vi "Main.vi"() -> ()   [LabVIEW 2013]
doc: "Configures a sweep and takes voltage and current readings at each point."
uses:
  <instrlib>/Keithley 24XX/Public/Data/Read (Multiple Points).vi
  <vilib>/Utility/file.llb/Read From Spreadsheet File (DBL).vi
  <instrlib>/Keithley 24XX/Keithley 24XX.lvlib
  <vilib>/gmath/NI_Gmath.lvlib
panel:
  in  "定标文件":string(combo)
  in  "Source Mode  (0: Voltage)":u16(ring) items=["Voltage", "Current"]
  in  "Serial Configuration":T1={"Baud Rate"=9600, "Parity"=0, "Data Bits"=8, "Stop Bits"=10, "Flow Control"=0} {"Flow Control" items=["None", "XON/XOFF", "RTS/CTS", "XON/XOFF & RTS/CTS", "DTR/DSR", "XON/XOFF & DTR/DSR"]; "Stop Bits" items=["1.0"=10, "1.5"=15, "2.0"=20]; "Data Bits" items=["7"=7, "8"=8]; "Parity" items=["None", "Odd", "Even", "Mark", "Space"]; "Baud Rate" items=["300"=300, "600"=600, "1200"=1200, "2400"=2400, "4800"=4800, "9600"=9600, "19200"=19200]}
  in  "VISA resource name":refnum<visa-resource-name>
  out "Waveform Graph":dbl[](graph)
  in  "Timeout (10000 ms)":i32=10000 format="%#.6g"
  in  "Maximum Amplitude (2)":dbl=2.0
  in  "Minimum Amplitude (1)":dbl=1.0
  in  "Number of Points (5)":u32=5
  in  "Compliance  Level (0.1)":dbl=0.1
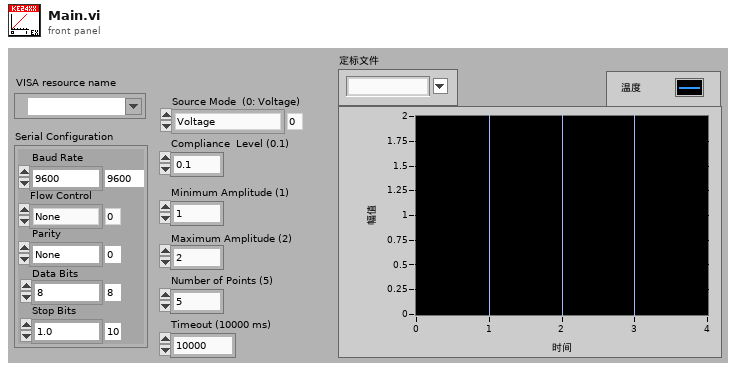
[diagram p1: front panel]
types:
  T1 = cluster{"Baud Rate":u32, "Parity":u16, "Data Bits":u16, "Stop Bits":u16, "Flow Control":u16}
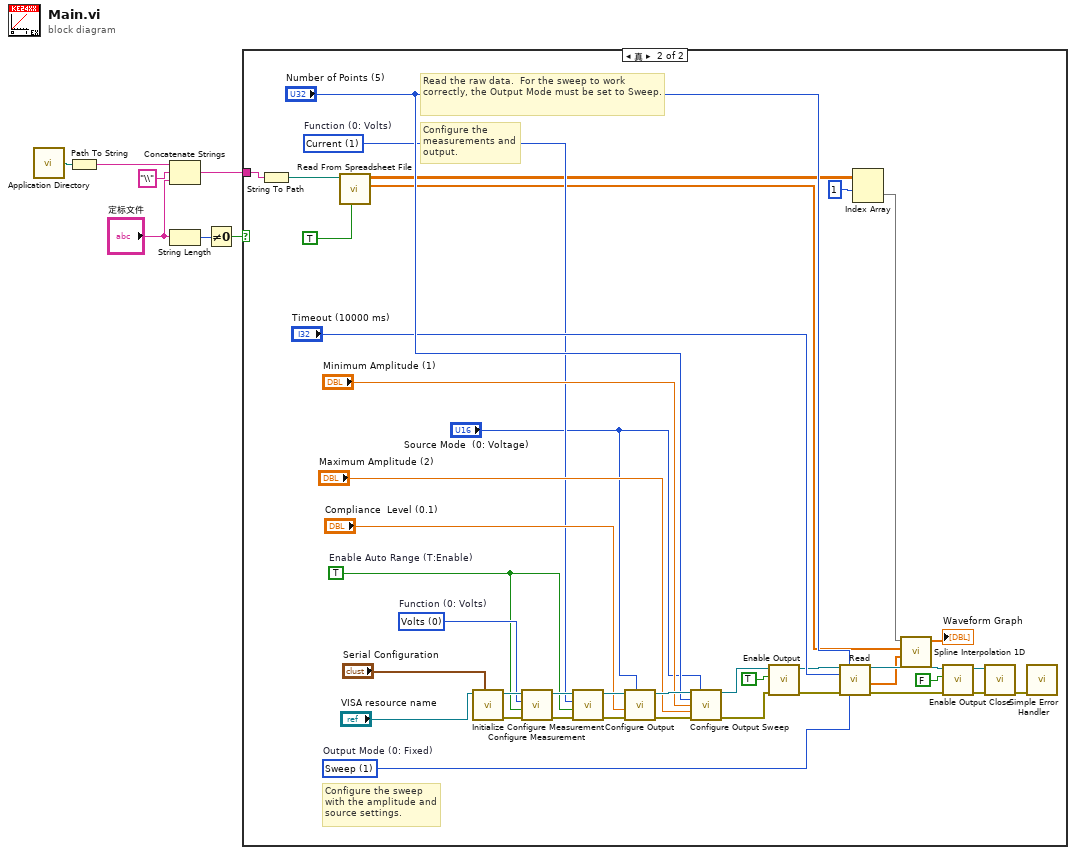
[diagram p0: block diagram]
diagram:
  n1 = call <vilib>:"Application Directory.vi"() -> ("Application Directory"=w7:path)
  n2 = Path To String(path=w7) -> (string=w6:string)
  n3 = Concatenate Strings(w6, "\\", "定标文件") -> (w2:string)
  n4 = String Length(string="定标文件") -> (length=w3:i32)
  n5 = Not Equal To 0?(x=w3) -> (x != 0?=w1:bool)
  n6 = case shown="真" w1 {
    tunnel: w2 -> [_ w9]
    frame False {
    }
    frame True {
      w19 = TRUE  # Enable Auto Range (T:Enable)
      w20 = u16 1 items=["Volts", "Current", "Resistance"]  # Function (0: Volts)
      w21 = u16 0 items=["Volts", "Current", "Resistance"]  # Function (0: Volts)
      w33 = u16 1 items=["Fixed", "Sweep", "List"]  # Output Mode (0: Fixed)
      # "Read the raw data.  For the sweep to work correctly, the Output Mode must be set to Sweep."
      # "Configure the sweep with the amplitude and source settings."
      # "Configure the measurements and output."
      n7 = String To Path(string=w9) -> (path=w8:path)
      n8 = call-poly <vilib>:"Read From Spreadsheet File.vi"("transpose (no:F)"=TRUE, "file path (dialog if empty)"=w8) -> ("first row"=w12:dbl[], "all rows"=w11:dbl[][])  [unwired: 5 in, 3 out]
      n9 = call <instrlib>:"Initialize.vi"("Serial Configuration"="Serial Configuration", "VISA resource name"="VISA resource name") -> ("error out"=w46:errorcluster, "VISA resource name out"=w47:refnum<visa-resource-name>)  [unwired: 8 in]
      n10 = call <instrlib>:"Configure Measurement.vi"("error in (no error)"=w46, "Enable Auto Range (T:Enable)"=w19, "Function (0: Volts)"=w21, "VISA resource name"=w47) -> ("error out"=w45:errorcluster, "VISA resource name out"=w44:refnum<visa-resource-name>)  [unwired: 6 in]
      n11 = call <instrlib>:"Configure Measurement.vi"("error in (no error)"=w45, "Enable Auto Range (T:Enable)"=w19, "Function (0: Volts)"=w20, "VISA resource name"=w44) -> ("error out"=w42:errorcluster, "VISA resource name out"=w43:refnum<visa-resource-name>)  [unwired: 6 in]
      n12 = call <instrlib>:"Configure Output.vi"("Source Mode  (0: Voltage)"="Source Mode  (0: Voltage)", "error in (no error)"=w42, "Compliance  Level (0.1)"="Compliance  Level (0.1)", "VISA resource name"=w43) -> ("error out"=w41:errorcluster, "VISA resource name out"=w40:refnum<visa-resource-name>)  [unwired: 6 in]
      n13 = call <instrlib>:"Configure Output Sweep.vi"("VISA resource name"=w40, "Source Mode  (0: Voltage)"="Source Mode  (0: Voltage)", "Number of Points (5)"="Number of Points (5)", "Minimum Amplitude (1)"="Minimum Amplitude (1)", "Maximum Amplitude (2)"="Maximum Amplitude (2)", "error in (no error)"=w41) -> ("VISA resource name out"=w24:refnum<visa-resource-name>, "error out"=w23:errorcluster)  [unwired: 8 in]
      n14 = call <instrlib>:"Enable Output.vi"("error in (no error)"=w23, "Enable Output (T: Enable)"=TRUE, "VISA resource name"=w24) -> ("error out"=w26:errorcluster, "VISA resource name out"=w25:refnum<visa-resource-name>)  [unwired: 7 in]
      n15 = call-poly <instrlib>:"Read.vi"("VISA resource name"=w25, "Sample Count (1)"="Number of Points (5)", "Timeout (10000 ms)"="Timeout (10000 ms)", "error in (no error)"=w26, "Output Mode (0: Fixed)"=w33) -> ("VISA resource name out"=w28:refnum<visa-resource-name>, "Resistance"=w14:sgl[], "error out"=w29:errorcluster)  [unwired: 4 in, 4 out]
      n16 = Index Array(array=w11, index (row)=1) -> (element=w15:dbl[])  [unwired: 1 in]
      n17 = call <vilib>:"Spline Interpolation 1D.vi"("xi"=w14, "X"=w12, "Y"=w15) -> ("yi"=→"Waveform Graph":dbl[])  [unwired: 6 in, 2 out]
      n18 = call <instrlib>:"Enable Output.vi"("error in (no error)"=w29, "Enable Output (T: Enable)"=FALSE, "VISA resource name"=w28) -> ("error out"=w30:errorcluster, "VISA resource name out"=w31:refnum<visa-resource-name>)  [unwired: 7 in]
      n19 = call <instrlib>:"Close.vi"("error in (no error)"=w30, "VISA resource name"=w31) -> ("error out"=w32:errorcluster)  [unwired: 9 in]
      n20 = call <vilib>:"Simple Error Handler.vi"("error in (no error)"=w32) -> ()  [unwired: 4 in, 5 out]
    }
  }
